vi "Set Alias.vi"(8 "error in (no error)":errorcluster, 10 "Alias":string, 11 "Device in":refnum<class "Device.lvclass">) -> (0 "error out":errorcluster, 3 "Device out":refnum<class "Device.lvclass">)   [LabVIEW 2020, in "PicoG-App.lvlib" / "Device.lvclass"]
uses:
  Device.lvclass
  Device.lvclass/Device.ctl
  Builds/picoG/ppl/PicoG-Core.lvlibp/PicoG-Processor/PicoG-Core/Resource/Resource.lvclass
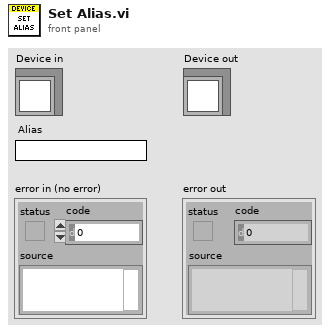
[diagram p1: front panel]
types:
  T1 = typedef "PicoG-App.lvlib/Device.lvclass/Ref Data.ctl" = cluster{"Alias":string, "Version":string, "Build":timestamp, "Key":T2}
  T2 = typedef "PicoG-App.lvlib/Device.lvclass/Device Key.ctl" = cluster{"Platform":string, "Board":string, "ID":string}
  T3 = typedef "PicoG-App.lvlib/Device.lvclass/Resource Ref.ctl" = cluster{"Resource":refnum<class "Resource.lvclass">, "Open":bool, "At Prompt":bool, "Running":bool}
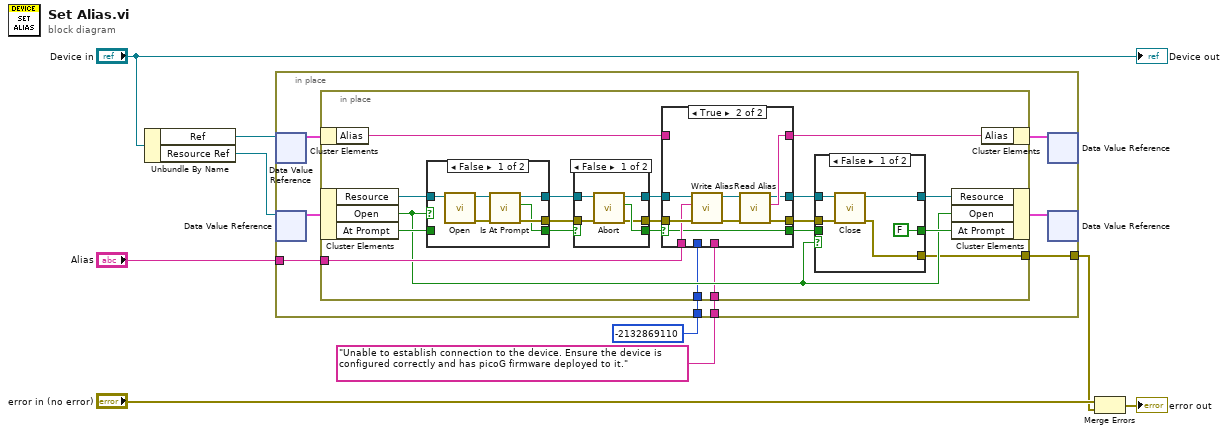
[diagram p0: block diagram]
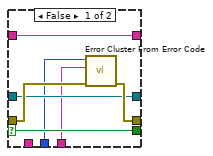
[diagram p5: hidden frame]
diagram:
  n1 = Unbundle By Name("Device in") -> ("Ref"=w7:refnum<data-value>, "Resource Ref"=w6:refnum<data-value>)
  n2 = in-place {
    in-place-border: "Alias" -> [w15]
    in-place-border: -2132869110 -> [w12]
    in-place-border: "Unable to establish connection to the device. Ensure the device is configured correctly and has picoG firmware deployed to it." -> [w11]
    in-place-border: [w10] -> w1
    n3 = in-place-dvr #1(w7) -> (w17:T1)  [unwired: 1 out]
    n4 = in-place-dvr #2(w6) -> (w16:T3)  [unwired: 1 out]
    n5 = in-place {
      in-place-border: w15 -> [w35]
      in-place-border: w12 -> [w20]
      in-place-border: w11 -> [w19]
      in-place-border: [w18] -> w10
      n6 = in-place-cluster #3(w17) -> ("Alias"=w33:string)
      n7 = in-place-cluster #4(w16) -> ("Resource"=w36:refnum<class "Resource.lvclass">, "Open"=w21:bool, "At Prompt"=w37:bool)
      n8 = case shown="False" w21 {
        tunnel: w37 -> [_ w53]
        tunnel: [w46 w53] -> w26
        tunnel: w36 -> [w51 w52]
        tunnel: [w49 w52] -> w27
        tunnel: [w47 _] -> w25
        frame False {
          n9 = call-dynamic "Open.vi"("DeployResource in"=w51) -> ("error out"=w48:errorcluster, "DeployResource out"=w50:refnum<class "Resource.lvclass">)  [unwired: 9 in]
          n10 = call-dynamic "Is At Prompt.vi"("error in (no error)"=w48, "DeployResource in"=w50) -> ("error out"=w47:errorcluster, "At Prompt?"=w46:bool, "DeployResource out"=w49:refnum<class "Resource.lvclass">)  [unwired: 6 in, 1 out]
        }
        frame True {
        }
      }
      n11 = case shown="False" w26 {
        selector: w26 -> [_ w45]
        tunnel: [w40 w45] -> w23
        tunnel: w27 -> [w42 w44]
        tunnel: [w39 w44] -> w22
        tunnel: w25 -> [w41 w43]
        tunnel: [w38 w43] -> w24
        frame False {
          n12 = call-dynamic "Abort.vi"("error in (no error)"=w41, "DeployResource in"=w42) -> ("error out"=w38:errorcluster, "Stopped?"=w40:bool, "DeployResource out"=w39:refnum<class "Resource.lvclass">)  [unwired: 6 in, 1 out]
        }
        frame True {
        }
      }
      n13 = case shown="True" w23 {
        selector: w23 -> [w64 w69]
        tunnel: w22 -> [w65 w77]
        tunnel: w24 -> [w68 w76]
        tunnel: w35 -> [_ w75]
        tunnel: [w66 w72] -> w34
        tunnel: w33 -> [w66 _]
        tunnel: [w65 w71] -> w32
        tunnel: [w67 w70] -> w31
        tunnel: [w64 w69] -> w29
        tunnel: w20 -> [w63 _]
        tunnel: w19 -> [w62 _]
        frame False {
          n14 = call <vilib>:"Error Cluster From Error Code.vi"("error in (no error)"=w68, "error message (\"\")"=w62, "error code (0)"=w63) -> ("error out"=w67:errorcluster)  [unwired: 6 in]
        }
        frame True {
          n15 = call "Write Alias.vi"("error in (no error)"=w76, "Alias"=w75, "DeployResource in"=w77) -> ("error out"=w73:errorcluster, "DeployResource out"=w74:refnum<class "Resource.lvclass">)  [unwired: 7 in]
          n16 = call "Read Alias.vi"("error in (no error)"=w73, "DeployResource in"=w74) -> ("error out"=w70:errorcluster, "Alias"=w72:string, "DeployResource out"=w71:refnum<class "Resource.lvclass">)  [unwired: 7 in]
        }
      }
      n17 = case shown="False" w21 {
        tunnel: w32 -> [w58 w60]
        tunnel: w31 -> [w57 w59]
        tunnel: [w56 w60] -> w30
        tunnel: w29 -> [_ w61]
        tunnel: [FALSE w61] -> w28
        tunnel: [w54 w59] -> w18
        frame False {
          n18 = call-dynamic "Close.vi"("error in (no error)"=w57, "DeployResource in"=w58) -> ("error out"=w54:errorcluster, "DeployResource out"=w56:refnum<class "Resource.lvclass">)  [unwired: 8 in]
        }
        frame True {
        }
      }
      n19 = in-place-cluster #4("Resource"=w30, "Open"=w21, "At Prompt"=w28) -> (w13:T3)
      n20 = in-place-cluster #3("Alias"=w34) -> (w14:T1)
    }
    n21 = in-place-dvr #1(w14) -> ()  [unwired: 2 out]
    n22 = in-place-dvr #2(w13) -> ()  [unwired: 2 out]
  }
  n23 = Merge Errors("error in (no error)", w1) -> (→"error out":errorcluster)
  "Device out" <- "Device in"
